vi "SLSC Session Property Node (Phys Chan).vi"   [LabVIEW 2020]
uses:
  <resource>/objmgr/slsc.rc
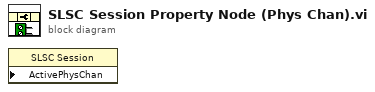
[diagram p0: block diagram]
diagram:
  n1 = property class="SLSC Session" props=["ActivePhysChan"]() -> ()  [unwired: 3 in, 2 out]
